vi "stepper pulsed.vi"() -> ()   [LabVIEW 2017]
uses:
  <vilib>/measure/NI_MABase.lvlib
panel:
  out "Stepper pulsed signal":waveform(dbl)[](graph)
  out "frequency":dbl
  in  "stop":bool
  in  "Current(A)":dbl
  in  "Speed(RPM)":dbl(knob) scale=0.0..100.0
  in  "Step Angle\n  (degree)":dbl
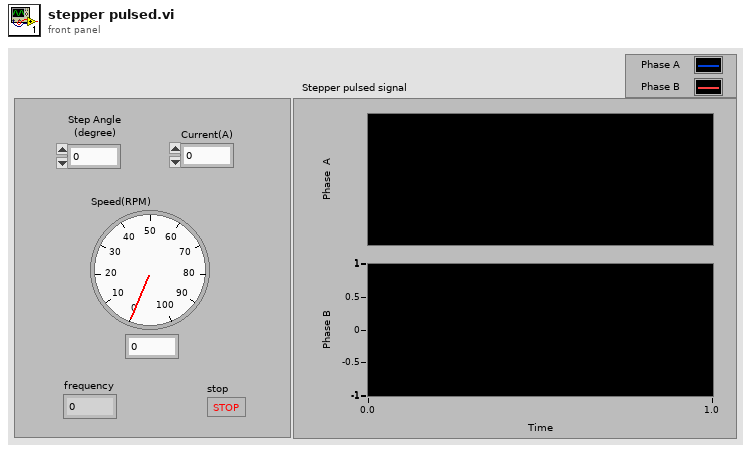
[diagram p1: front panel]
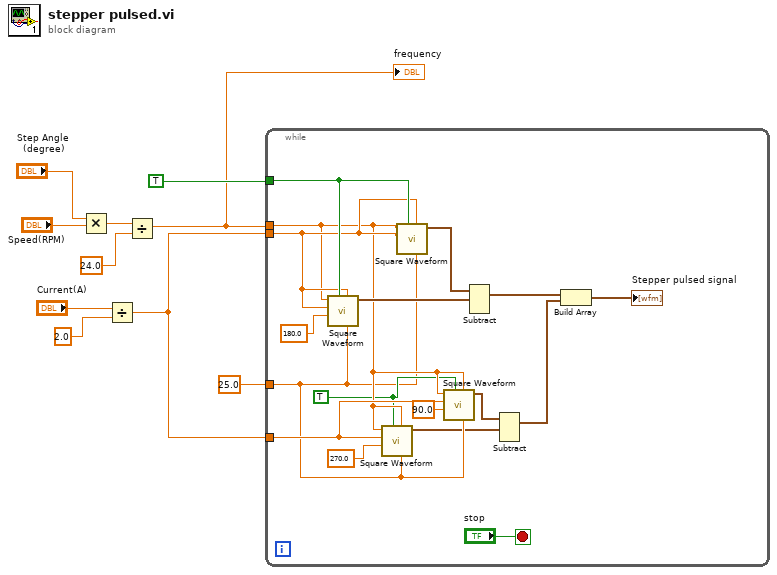
[diagram p0: block diagram]
diagram:
  n1 = Multiply(x="Step Angle\n  (degree)", y="Speed(RPM)") -> (x*y=w8:dbl)
  n2 = Divide(x="Current(A)", y=2.0) -> (x/y=w2:dbl)
  n3 = Divide(x=w8, y=24.0) -> (x/y=w1:dbl)
  "frequency" <- w1
  n4 = while {
    tunnel: w1 -> [w19]
    tunnel: w2 -> [w25]
    tunnel: 25.0 ("duty cycle (%)") -> [w17]
    tunnel: TRUE ("reset signal") -> [w26]
    tunnel: w2 -> [w20]
    stop <- "stop" stop-if-true
    w18 = TRUE ("reset signal")
    n5 = call <vilib>:"Square Waveform.vi"("duty cycle (%)"=w17, "offset"=w25, "reset signal"=w26, "phase"=180.0, "amplitude"=w25, "frequency"=w19) -> ("signal out"=w23:waveform(dbl))  [unwired: 4 in, 1 out]
    n6 = call <vilib>:"Square Waveform.vi"("duty cycle (%)"=w17, "offset"=w19, "reset signal"=w18, "phase"=270.0, "amplitude"=w20, "frequency"=w19) -> ("signal out"=w15:waveform(dbl))  [unwired: 4 in, 1 out]
    n7 = call <vilib>:"Square Waveform.vi"("duty cycle (%)"=w17, "offset"=w25, "reset signal"=w26, "amplitude"=w25, "frequency"=w19) -> ("signal out"=w22:waveform(dbl))  [unwired: 5 in, 1 out]
    n8 = call <vilib>:"Square Waveform.vi"("duty cycle (%)"=w17, "offset"=w19, "reset signal"=w18, "phase"=90.0, "amplitude"=w20, "frequency"=w19) -> ("signal out"=w14:waveform(dbl))  [unwired: 4 in, 1 out]
    n9 = Subtract(1:w23, 2:w22) -> (0:w13:waveform(dbl))  [unwired: 1 in, 1 out]
    n10 = Subtract(1:w15, 2:w14) -> (0:w12:waveform(dbl))  [unwired: 1 in, 1 out]
    n11 = Build Array(w13, w12) -> (→"Stepper pulsed signal":waveform(dbl)[])
  }
